vi "input registers fgv.vi"(7 "Action":T1, 8 "error in (no error)":errorcluster, 10 "RegisterMap in":T2[](array[typedef]) {"Address" format="%.0x"}) -> (0 "error out":errorcluster, 2 "RegisterMap out":T2[](array[typedef]) {"Address" format="%.0x"})   [LabVIEW 2016]
uses:
  <vilib>/rvi/Bitfile/nirviControlStructure.ctl
  <vilib>/rvi/Bitfile/nirviTypdefDescription.ctl
  <vilib>/rvi/Bitfile/nirviMechanicalAction.ctl
  <vilib>/rvi/Bitfile/nirviSubControlStructure.ctl
  <vilib>/rvi/Bitfile/nirviClusterElementControl.ctl
  Shared/FG Action.ctl
  Shared/FPGA Addon Shared.lvlib
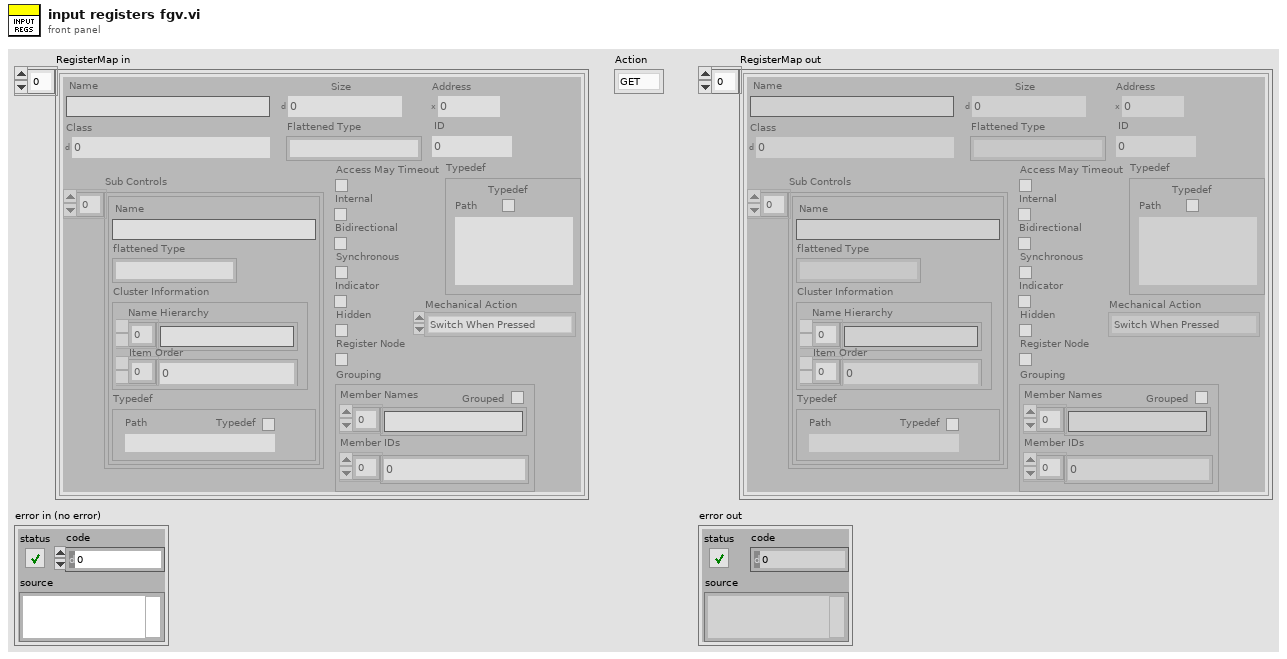
[diagram p1: front panel]
types:
  T1 = typedef "FPGA Addon Shared.lvlib/FG Action.ctl" = enum8{"GET", "SET"}
  T2 = typedef "nirviControlStructure.ctl" = cluster{"Name":string, "Hidden":bool, "Indicator":bool, "Flattened Type":string, "Grouping":cluster{"Grouped":bool, "Member Names":string[], "Member IDs":u32[]}, "Address":u32, "Size":u32, "Class":u32, "Internal":bool, "Typedef":T3, "ID":u32, "Bidirectional":bool, "Synchronous":bool, "Mechanical Action":T4, "Sub Controls":T5[], "Access May Timeout":bool, "Register Node":bool}
  T3 = typedef "nirviTypdefDescription.ctl" = cluster{"Typedef":bool, "Path":path}
  T4 = typedef "nirviMechanicalAction.ctl" = enum8{"Switch When Pressed", "Switch When Released", "Switch Until Released", "Latch When Pressed", "Latch When Released", "Latch Until Released"}
  T5 = typedef "nirviSubControlStructure.ctl" = cluster{"Name":string, "flattened Type":string, "Cluster Information":T6, "Typedef":T3}
  T6 = typedef "nirviClusterElementControl.ctl" = cluster{"Name Hierarchy":string[], "Item Order":u32[]}
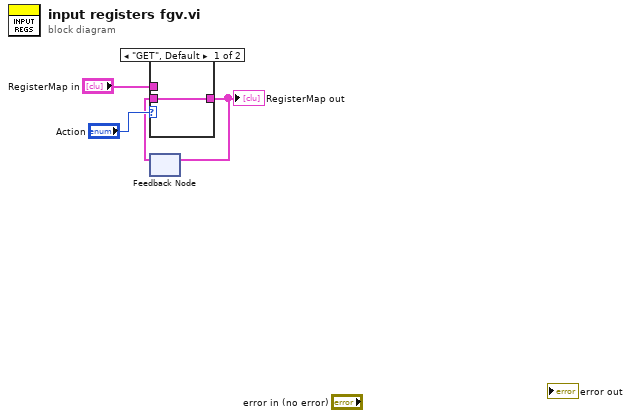
[diagram p0: block diagram]
diagram:
  n1 = feedback #1() -> (w1:T2[])  [unwired: 1 in]
  n2 = case shown="\"GET\", Default" "Action" {
    tunnel: w1 -> [w5 _]
    tunnel: [w5 w6] -> w3
    tunnel: "RegisterMap in" -> [_ w6]
    frame "GET", Default {
    }
    frame "SET" {
    }
  }
  "RegisterMap out" <- w3
  n3 = feedback-in #1(w3) -> ()
